vi "Accelration Control (by Throttle).vi"(3 "acc":dbl, 4 "input":dbl) -> (1 "output":dbl format="%.2f")   [LabVIEW 2011]
uses:
  <vilib>/addons/control/pid/pid.llb/PID Control Input Filter (DBL).vi
  <vilib>/addons/control/pid/pid.llb/PID Output Rate Limiter (DBL).vi
  <vilib>/addons/control/pid/NI_PID_pid.lvlib
  <vilib>/addons/control/pid/pid.llb/PID Lead-Lag (DBL).vi
panel:
  in  "fNode":dbl
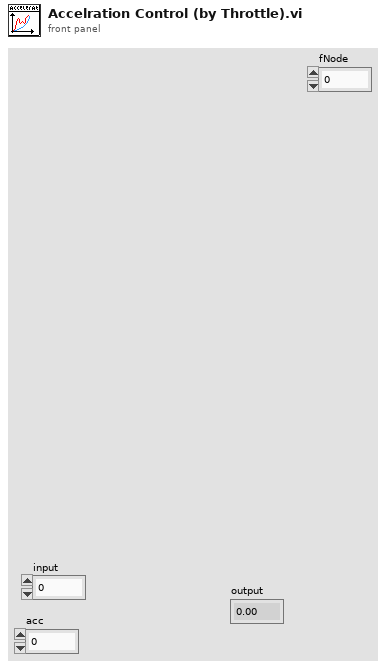
[diagram p1: front panel]
types:
  T1 = cluster{"gain":dbl, "lag time (min)":dbl, "lead time (min)":dbl}
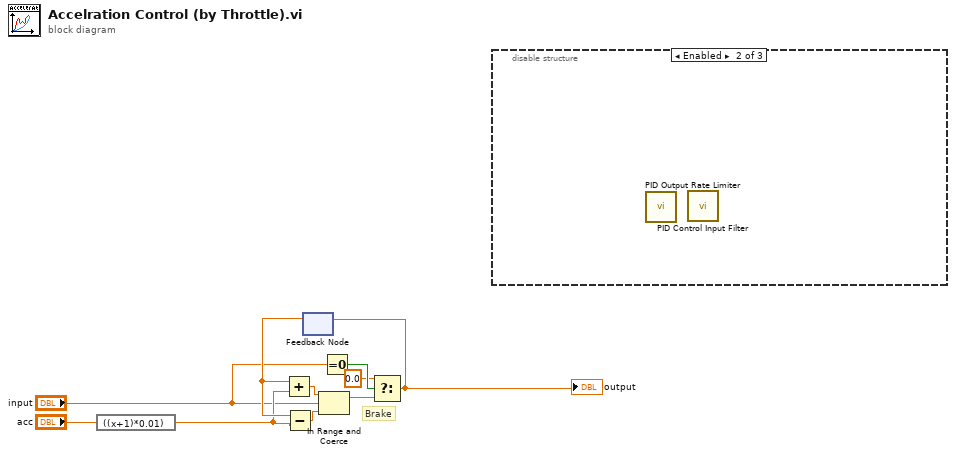
[diagram p0: block diagram]
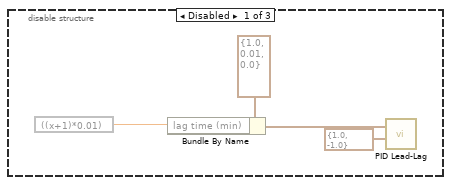
[diagram p2: hidden frame]
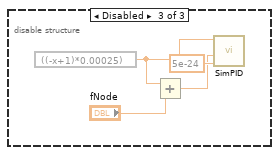
[diagram p3: hidden frame]
diagram:
  # "Brake"
  n1 = expression code="((x+1)*0.01)"("acc") -> (w6:dbl)
  n2 = feedback #1() -> (w8:dbl)  [unwired: 1 in]
  n3 = Add(x=w8, y=w6) -> (x+y=w9:dbl)
  n4 = Subtract(x=w8, y=w6) -> (x-y=w10:dbl)
  n5 = In Range and Coerce(upper limit=w9, x="input", lower limit=w10) -> (coerced(x)=w3:dbl)  [unwired: 1 out]
  n6 = Equal To 0?(x="input") -> (x = 0?=w4:bool)
  n7 = Select(t=0.0, s=w4, f=w3) -> (s? t:f=w1:dbl)
  "output" <- w1
  n8 = feedback-in #1(w1) -> ()
  n9 = disable-structure shown="Enabled" {
    frame Disabled {
      n10 = expression code="((x+1)*0.01)"() -> (w15:dbl)  [unwired: 1 in]
      n11 = Bundle By Name(cluster=T1 {"gain"=1.0, "lag time (min)"=0.01, "lead time (min)"=0.0} ("tuning parameters"), "lag time (min)"=w15) -> (w14:T1)
      n12 = call-poly <vilib>:"PID Lead-Lag.vi"("output range"=cluster{"output high":dbl, "output low":dbl} {"output high"=1.0, "output low"=-1.0}, "tuning parameters"=w14) -> ("output"=w12:dbl, "reinitialize? (F)"=w13:bool, "input"=w11:dbl)  [unwired: 2 in, 3 out]
    }
    frame Enabled {
      n13 = call-poly <vilib>:"PID Output Rate Limiter.vi"() -> ()  [unwired: 8 in, 2 out]
      n14 = call-poly <vilib>:"PID Control Input Filter.vi"() -> ()  [unwired: 5 in, 1 out]
    }
    frame Disabled {
      n15 = expression code="((-x+1)*0.00025)"() -> (w20:dbl)  [unwired: 1 in]
      n16 = Add(x=w20, y="fNode") -> (x+y=w19:dbl)
      n17 = call "SimPID.vi"("Range"=5e-24, "Position"=w19, "Gain"=w20) -> ("result"=w21:dbl, "Set Point"=w22:dbl)  [unwired: 5 in, 1 out]
    }
  }
